vi "UI_1.vi"() -> (15 "Compressor  O/P":bool, 16 "Cond O/P":bool, 17 "Ev_Fan_1 O/P":bool, 18 "Ev_Fan_2 O/P":bool, 19 "Heater O/P":bool)   [LabVIEW 2017]
uses:
  Automatic_button.ctl
  Administration_button.ctl
  <vilib>/Utility/miscctls.llb/LVAnnotationListTypeDef.ctl
  admin_settings.vi
  <vilib>/Utility/file.llb/Write Delimited Spreadsheet (DBL).vi
  <vilib>/Utility/file.llb/Write Delimited Spreadsheet (string).vi
  <vilib>/Utility/NIReport.llb/NI_report.lvclass
  <resource>/objmgr/daqmx.rc
  <vilib>/Utility/NIReport.llb/Append Image to Report (path wrap).vi
  <vilib>/Utility/NIReport.llb/Append Text Table to Report (wrap).vi
panel:
  out "DevSerialNum 2":u32
  out "DevSerialNum":u32
  out "error out 6":errorcluster
  out "error out 11":errorcluster
  out "error out 10":errorcluster
  out "error out 9":errorcluster
  out "error out 8":errorcluster
  out "error out 7":errorcluster
  out "error out 4":errorcluster
  out "error out 3":errorcluster
  out "error out 5":errorcluster
  out "error out 2":errorcluster
  out "error out":errorcluster
  in  "Conrtols AUX 3":T1
  in  "Conrtols Valves 2":T2
  out "NI2":tag
  out "NI1":tag
  in  "Conrtols AUX 2":T1
  in  "Conrtols Valves":T2
  in  "Tab Control":enum32{"System", "Charts", "Faults"}(tab)
  out "Testing Mode":bool
  in  "Administration":T3
  in  "set point R":dbl
  in  "set point F":dbl
  in  "Auto":T4
  in  "Exit":bool
  out "T 9":dbl format="%#_3g"
  out "Segemnt_1.1 6":bool
  out "?":bool
  out "3.30":bool
  out "?":bool
  out "?":bool
  in  "Valve_8":bool
  in  "Valve_9":bool
  in  "Valve_10":bool
  out "T 4":dbl format="%#_3g"
  in  "Valve_2":bool
  out "P1":dbl format="%#_3g"
  out "T1":dbl format="%#_3g"
  out "S3.12":bool
  in  "Valve_11":bool
  out "T 10":dbl format="%#_3g"
  out "T 11":dbl format="%#_3g"
  out "P 3":dbl format="%#_3g"
  out "T 3":dbl format="%#_3g"
  out "S3.27":bool
  out "S3.23":bool
  out "S3.19":bool
  out "S3.28":bool
  out "S3.16":bool
  out "S3.18":bool
  out "?":bool
  out "OK Button 16":bool
  out "S3.15":bool
  out "?":bool
  out "?":bool
  out "?":bool
  out "Segment 1.4 5":bool
  out "?":bool
  out "?":bool
  in  "Ev_Fan_1":bool
  in  "Heater":bool
  in  "Valve_3":bool
  in  "Valve_4":bool
  in  "Valve_5":bool
  out "Segment_1":bool
  out "?":bool
  out "?":bool
  out "Segment_1 2":bool
  out "Segment 1.3":bool
  out "Segment 1.4":bool
  out "?":bool
  out "Segemnt_1.1 2":bool
  out "?":bool
  out "?":bool
  out "?":bool
  out "T 6":dbl format="%#_3g"
  out "?":bool
  out "OK Button":bool
  out "?":bool
  out "Segment 1.4 4":bool
  out "?":bool
  out "OK Button 3":bool
  out "Segemnt_1.1 3":bool
  out "?":bool
  out "OK Button 4":bool
  out "OK Button 5":bool
  out "OK Button 6":bool
  out "?":bool
  out "S3.37":bool
  out "S3.36":bool
  out "S3.35":bool
  out "Segment 1.4 7":bool
  out "?":bool
  out "?":bool
  in  "Ev_Fan_2":bool
  in  "Valve_6":bool
  in  "Valve_7":bool
  out "Segment_1 5":bool
  out "Segemnt_1.1 4":bool
  out "Segment_1 6":bool
  out "?":bool
  out "T 8":dbl format="%#_3g"
  out "?":bool
  out "Segemnt_1.1 5":bool
  out "?":bool
  out "?":bool
  out "?":bool
  out "T 7":dbl format="%#_3g"
  out "?":bool
  out "OK Button 11":bool
  out "?":bool
  out "Segment 1.4 8":bool
  out "?":bool
  out "OK Button 13":bool
  out "OK Button 15":bool
  out "?":bool
  out "P 4":dbl format="%#_3g"
  out "Segment_1 7":bool
  out "Segment_1 8":bool
  out "Segment_1 9":bool
  out "?":bool
  out "?":bool
  out "?":bool
  out "?":bool
  out "?":bool
  out "Segemnt_1.1 7":bool
  out "?":bool
  out "S3.1":bool
  out "S3.2":bool
  out "S3.3":bool
  out "S3.4":bool
  out "P5":dbl format="%#_3g"
  out "T5":dbl format="%#_3g"
  out "S3.6":bool
  out "S3.8":bool
  out "S3.11":bool
  out "S3.10":bool
  out "S3.9":bool
  out "S3.39":bool
  out "S3.38":bool
  out "?":bool
  out "3.34":bool
  out "3.33":bool
  out "3.32":bool
  out "?":bool
  out "3.31":bool
  out "?":bool
  out "S3.29":bool
  out "3.24":bool
  out "3.22":bool
  out "?":bool
  out "S3.25":bool
  out "3.21":bool
  out "3.20":bool
  out "Segment 1.4 2":bool
  out "Segment 1.4 3":bool
  in  "Cond":bool
  out "S3.14":bool
  out "S3.13":bool
  out "S3.17":bool
  in  "Valve_1":bool
  in  "Compressor":bool
  out "Segment 1.4 6":bool
  out "Segment 1.4 9":bool
  out "P 2":dbl format="%#_3g"
  out "T 2":dbl format="%#_3g"
  out "?":bool
  out "?":bool
  out "S3.25 2":bool
  out "?":bool
  out "S3.7":bool
  out "S3.5":bool
  in  "Save table":bool
  in  "Save image":bool
  in  "Tab Control 2":T5(tab)
  out "Cycle 1":string="6 ==> T11 , P11\n1 ==> T5 , P5\n2 ==> T1 , P1\n3 ==> T2 , P2\n4 ==> T9 , P2\n5 ==> T3 , P3"
  out "Cycle 2":string="6 ==> T11 , P11\n1 ==> T5 , P5\n2 ==> T1 , P1\n3 ==> T2 , P2\n4 ==> T9 , P2\n5 ==> T3 , P3"
  out "Cycle 3":string="6 ==> T11 , P11\n1 ==> T5 , P5\n2 ==> T1 , P1\n3 ==> T2 , P2\n4 ==> T9 , P2\n5 ==> T3 , P3"
  out "Cycle 4":string="9 ==> T10 , P10\n1 ==> T5 , P5\n2 ==> T1 , P1\n3 ==> T2 , P2\n7 ==> T8 , P2\n8 ==> T4 , P4"
  out "Cycle 5":string="9 ==> T10 , P10\n1 ==> T5 , P5\n2 ==> T1 , P1\n3 ==> T2 , P2\n7 ==> T8 , P2\n8 ==> T4 , P4"
  out "Cycle 6":string="9 ==> T10 , P10\n1 ==> T5 , P5\n2 ==> T1 , P1\n3 ==> T2 , P2\n7 ==> T8 , P2\n8 ==> T4 , P4"
  out "Cycle 7":string="1 ==> T5 , P5\n2 ==> T1 , P1\n3 ==> T2 , P2\n7 ==> T8 , P2\n8 ==> T4 , P4\n9 ==> T10 , P10\n\n4 ==> T9 , P2\n5 ==> T3 , P3\n6 ==> T11 , P11"
  out "Cycle 8":string="1 ==> T5 , P5\n2 ==> T1 , P1\n3 ==> T2 , P2\n7 ==> T8 , P2\n8 ==> T4 , P4\n9 ==> T10 , P10\n\n4 ==> T9 , P2\n5 ==> T3 , P3\n6 ==> T11 , P11"
  out "Cycle 9":string="1 ==> T5 , P5\n2 ==> T1 , P1\n3 ==> T2 , P2\n7 ==> T8 , P2\n8 ==> T4 , P4\n9 ==> T10 , P10\n\n4 ==> T9 , P2\n5 ==> T3 , P3\n6 ==> T11 , P11"
  out "Performance parameters":T6
  in  "Draw Points 2":bool
  out "Table":string[][](table)
  in  "Cycle":string(combo)="Cycle 1"
  in  "Draw Points":bool
  out "XY Graph":cluster{"all rows":dbl[], "all rows":dbl[]}[](graph)
  in  "m_dot_total":dbl=2.0 format="%#_13g"
  in  "m_dot_1":dbl=1.0 format="%#_13g"
  in  "m_dot_2":dbl=1.0 format="%#_13g"
  in  "h":dbl=372.0 format="%#_13g"
  in  "Valve 15 Fault":bool
  in  "Valve 13 Fault":bool
  in  "Valve 12 Fault":bool
  in  "Valve 11 Fault":bool
  # "TC"
  # "TC"
  # "Kg/s"
  # "KJ/Kg"
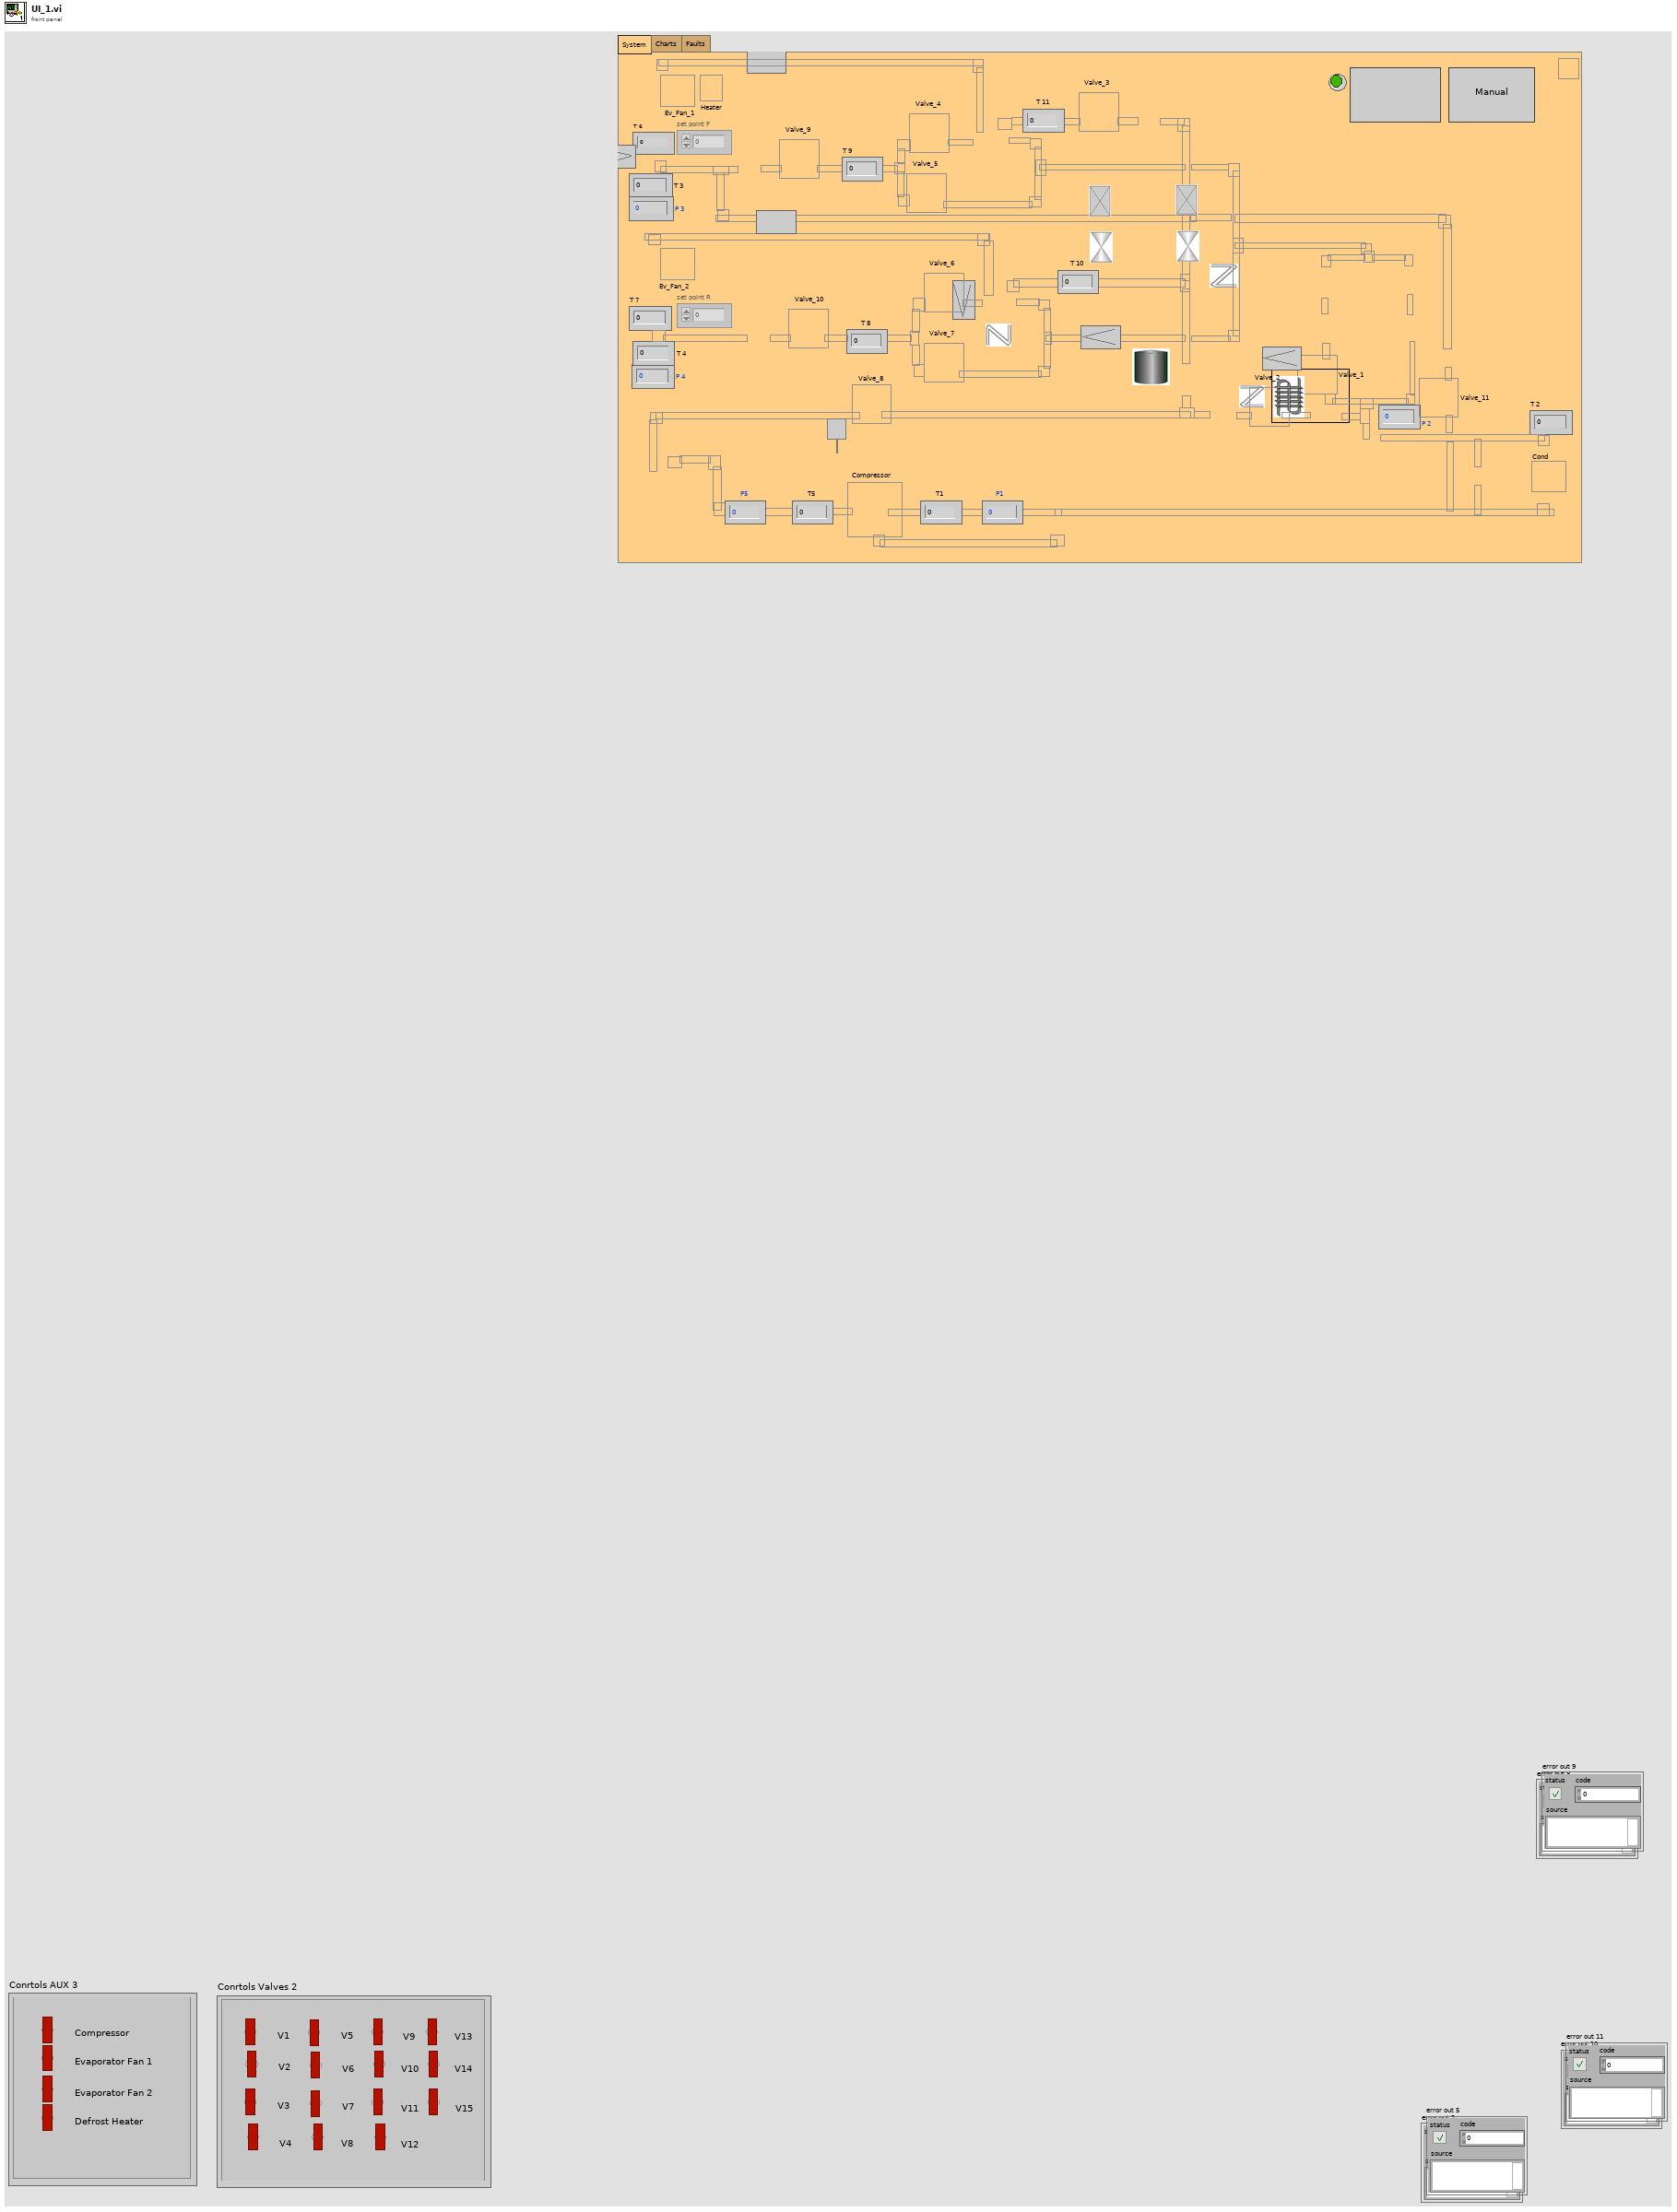
[diagram p1: front panel]
types:
  T1 = cluster{"Compressor":bool, "Evaporator Fan 1":bool, "Evaporator Fan 2":bool, "Defrost Heater":bool}
  T2 = cluster{"V1":bool, "V2":bool, "V3":bool, "V4":bool, "V5":bool, "V6":bool, "V7":bool, "V8":bool, "V9":bool, "V10":bool, "V11":bool, "V12":bool, "V13":bool, "V14":bool, "V15":bool}
  T3 = typedef "Administration_button.ctl" = bool
  T4 = typedef "Automatic_button.ctl" = bool
  T5 = enum32{"1", "2", "3", "4", "5", "6", "7", "8", "9"}
  T6 = cluster{"Condensation Capacity":dbl, "C.O.P  freez":dbl, "C.O.P  refrig":dbl}
  T7 = typedef "LVAnnotationListTypeDef.ctl" = cluster{"Name":string, "Color":u32, "Style":u8, "Point Style":u8, "Name Visible":bool, "Allow Drag":bool, "Annotation Mode":u32, "Plot":i32, "Index":i32, "Position":cluster{"X":dbl, "Y":dbl}, "X Scale":u32, "Y Scale":u32, "Show Arrow":bool, "Lock Name":bool, "Plot Area":i32, "Label Offset":cluster{"X":dbl, "Y":dbl}}[]
  T8 = enum16{"Standard Report", "HTML", "Word", "Excel"}
  T9 = enum8{"Enabled", "Disabled", "Disabled and Grayed Out"}
  T10 = cluster{"P1":dbl, "P2":dbl, "P3":dbl, "P4":dbl, "P5":dbl}
  T11 = cluster{"T1":dbl, "T2":dbl, "T3":dbl, "T4":dbl, "T5":dbl, "T6":dbl, "T7":dbl, "T8":dbl, "T9":dbl, "T10":dbl, "T11":dbl}
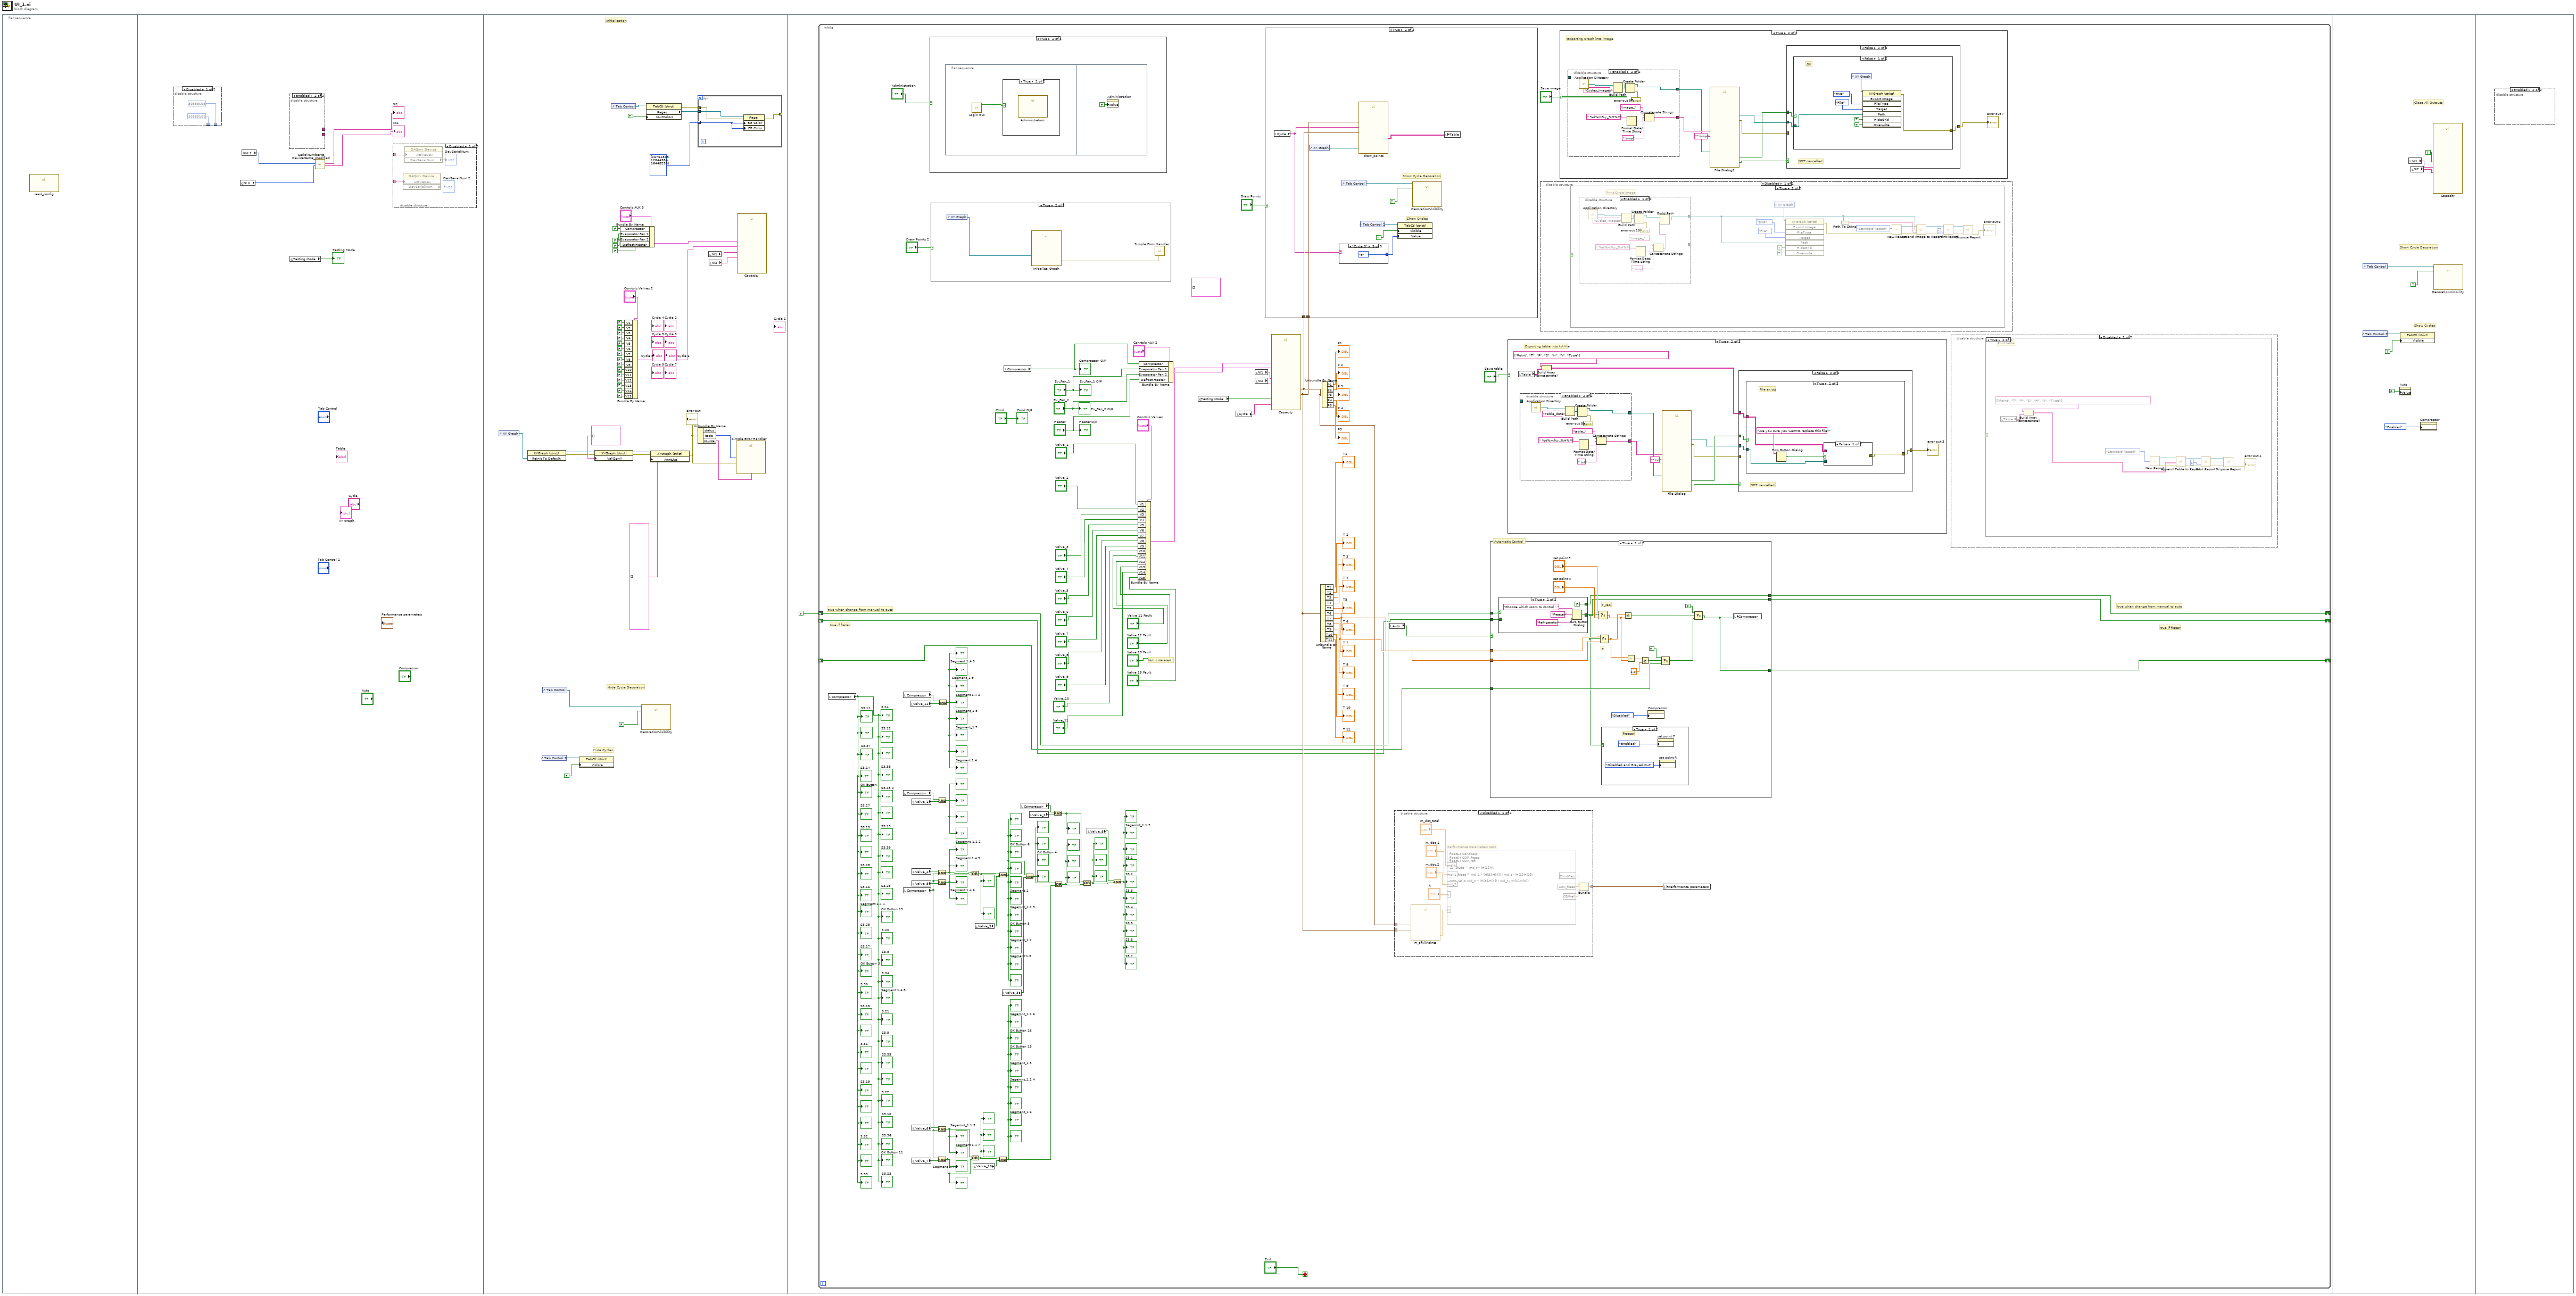
[diagram p0: block diagram]
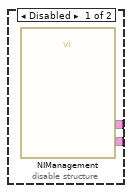
[diagram p4: hidden frame]
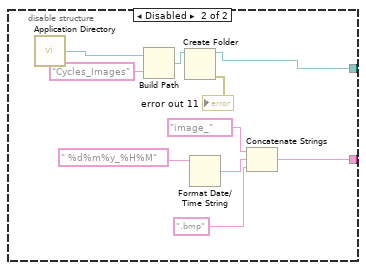
[diagram p8: hidden frame]
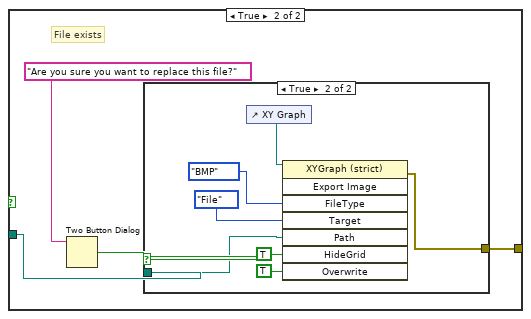
[diagram p14: hidden frame]
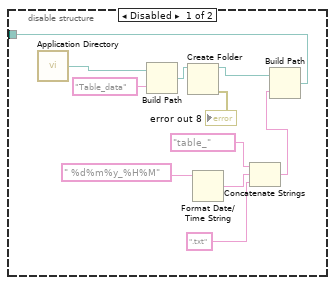
[diagram p16: hidden frame]
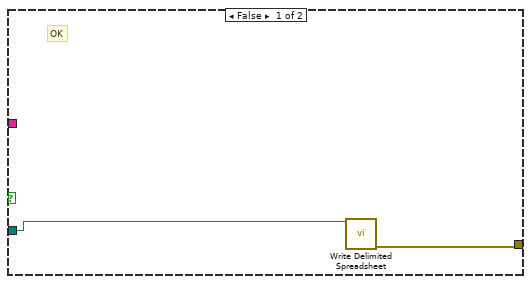
[diagram p19: hidden frame]
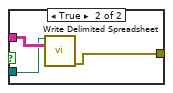
[diagram p20: hidden frame]
diagram:
  n1 = flat-sequence {
    frame #0 {
      n2 = call "read_config.vi"() -> ()  [unwired: 12 in]
    }
    frame #1 {
      n3 = disable-structure shown="Disabled" {
        disable-tunnel: [i64 30585608 ("NI1 Serial Number") _] -> _
        disable-tunnel: [i64 30585101 ("NI2 Serial Number") _] -> _
        frame Disabled {
        }
        frame Enabled {
        }
      }
      n4 = global read "admin_settings.vi" "NI 2"() -> (w3:i64)
      n5 = global read "admin_settings.vi" "NI 1"() -> (w4:i64)
      n6 = disable-structure shown="Enabled" {
        disable-tunnel: [w13 _] -> _
        disable-tunnel: [w12 _] -> _
        frame Disabled {
          n7 = call "NIManagement.vi"() -> ("NI2"=w12:tag, "NI1"=w13:tag)  [unwired: 8 in, 2 out]
        }
        frame Enabled {
        }
      }
      n8 = global read "admin_settings.vi" "Testing Mode"() -> (→"Testing Mode":bool)
      n9 = call "SerialNumber to DeviceName_modified.vi"("NI2 Serial Number"=w3, "NI1 Serial Number"=w4) -> ("NI2 Device Name"=→"NI2":tag, "NI1 Device Name"=→"NI1":tag)  [unwired: 7 in, 1 out]
      n10 = disable-structure shown="Disabled" {
        disable-tunnel: _ -> [w7 _]
        disable-tunnel: _ -> [w6 _]
        frame Disabled {
          n11 = property class="DAQmx Device"("ActiveDev"=w6) -> ("DevSerialNum"=→"DevSerialNum 2":u32)  [unwired: 2 in, 2 out]
          n12 = property class="DAQmx Device"("ActiveDev"=w7) -> ("DevSerialNum"=→"DevSerialNum":u32)  [unwired: 2 in, 2 out]
        }
        frame Enabled {
        }
      }
    }
    frame #2 {
      # "Hide Cycles"
      # "Hide Cycle Decoration"
      # "Initialization"
      n13 = control-ref of="XY Graph"() -> (w20:refnum<vi>)
      n14 = invoke class="XYGraph (strict)" method="Reinit To Default"(reference=w20) -> (reference out=w26:refnum<vi>, error out=w17:errorcluster)  [unwired: 2 in, 1 out]
      n15 = control-ref of="Tab Control 2"() -> (w15:refnum<vi>)
      n16 = control-ref of="Tab Control"() -> (w19:refnum<vi>)
      n17 = property class="TabCtl (strict)"(reference=w15, "Visible"=FALSE) -> ()  [unwired: 1 in, 2 out]
      n18 = property class="XYGraph (strict)"(reference=w26, error in=w17, "Val(Sgnl)"=cluster{"all rows":dbl[], "all rows":dbl[]}[] [] ("Value (Signaling)")) -> (reference out=w25:refnum<vi>, error out=w23:errorcluster)
      n19 = control-ref of="Tab Control"() -> (w28:refnum<vi>)
      n20 = Bundle By Name(cluster="Conrtols AUX 3", "Compressor"=FALSE, "Evaporator Fan 1"=FALSE, "Evaporator Fan 2"=FALSE, "Defrost Heater"=FALSE) -> (w36:T1)
      n21 = Bundle By Name(cluster="Conrtols Valves 2", "V1"=FALSE, "V2"=FALSE, "V3"=FALSE, "V4"=FALSE, "V5"=FALSE, "V6"=FALSE, "V7"=FALSE, "V8"=FALSE, "V9"=FALSE, "V10"=FALSE, "V11"=FALSE, "V12"=FALSE, "V13"=FALSE, "V14"=FALSE, "V15"=FALSE) -> (w35:T2)
      n22 = call "DecorationVisibility.vi"("Visible"=FALSE, "TabControl in"=w19) -> ()  [unwired: 9 in, 1 out]
      n23 = property class="TabCtl (strict)"(reference=w28, "MultColors"=TRUE ("Mehrere Farben zulassen")) -> (error out=w30:errorcluster, "Pages"=w32:refnum<vi>[])  [unwired: 1 in, 1 out]
      n24 = property on="Property Node" class="XYGraph (strict)"(reference=w25, error in=w23, "AnntList"=T7 [] ("Annotation List")) -> (error out=w18:errorcluster)  [unwired: 1 out]
      "error out" <- w18
      n25 = for {
        tunnel: w32 -> [w61] mode=indexing
        tunnel: u32[] [16764808, 12844984, 16448250] -> [w60] mode=indexing
        tunnel: w30 -> [w59]
        tunnel: [w58] -> _ mode=indexing
        n26 = property class="Page"(reference=w61, error in=w59, "BG Color"=w60, "FG Color"=w60) -> (error out=w58:errorcluster)  [unwired: 1 out]
      }
      n27 = Unbundle By Name(w18) -> ("code"=w21:i32, "source"=w22:string)  [unwired: 1 out]
      n28 = local read "NI1"() -> (w34:tag)
      n29 = local read "NI2"() -> (w33:tag)
      n30 = call <vilib>:"Simple Error Handler.vi"("error code (no error:0)"=w21, "error source (\" \")"=w22, "error in (no error)"=w18) -> ()  [unwired: 2 in, 5 out]
      n31 = call "Capacity.vi"("Conrtols Valves"=w35, "Conrtols AUX"=w36, "NI1"=w34, "NI2"=w33) -> ()  [unwired: 10 in, 2 out]
    }
    frame #3 {
      n32 = while {
        shift-right: [w74] -> _
        shift-left: _ -> [w73]
        shift-right: [w70] -> _
        shift-left: TRUE -> [w71]
        shift-right: [w69] -> _
        shift-left: _ -> [w68]
        stop <- "Exit" stop-if-true
        (unwired) cluster{"all rows":dbl[], "all rows":dbl[]}[] [] ("Output Graphs")
        # "Automatic Control"
        # "true when change from manual to auto"
        # "true if frezer"
        # "true when change from manual to auto"
        # "true if frezer"
        # "Not is deleted !"
        n33 = local read "Compressor"() -> (→"S3.8" →"S3.9" →"S3.10" →"S3.11" →"S3.15" →"S3.19" →"S3.14" →"S3.16" →"S3.17" →"S3.18" →"S3.13" →"S3.12" →"3.22" →"S3.25 2" →"S3.23" →"3.21" →"3.20" →"S3.25" →"S3.29" →"3.33" →"3.30" →"S3.27" →"S3.28" →"3.34" →"?" →"S3.35" →"S3.39" →"S3.38" →"S3.37" →"3.32" →"S3.36" →"3.24" →"3.31" →"?" →"?" →"?" →"OK Button" →"?" →"Segment 1.4 4" →"?" →"OK Button 3" →"?" →"?" →"?" →"?" →"OK Button 13" →"Segment 1.4 8" →"OK Button 11" →"?":bool)
        n34 = local read "Compressor"() -> (w150:bool)
        n35 = local read "Compressor"() -> (w151:bool)
        n36 = local read "Compressor"() -> (w137:bool)
        n37 = local read "Valve_11"() -> (w149:bool)
        n38 = local read "Valve_1"() -> (w152:bool)
        n39 = local read "Valve_4"() -> (w145:bool)
        n40 = local read "Valve_5"() -> (w144:bool)
        n41 = local read "Valve_6"() -> (w139:bool)
        n42 = local read "Valve_7"() -> (w138:bool)
        n43 = case shown="True" "Administration" {
          frame False {
          }
          frame True {
            n44 = flat-sequence {
              frame #0 {
                n45 = call "Login GUI.vi"() -> ("true"=w154:bool)  [unwired: 11 in]
                n46 = case shown="True" w154 {
                  frame False {
                  }
                  frame True {
                    n47 = call "Administration.vi"() -> ()  [unwired: 12 in]
                  }
                }
              }
              frame #1 {
                n48 = property on="Administration" class="Bool (strict)"("Value"=T3 FALSE ("Administration")) -> ()  [unwired: 2 in, 2 out]
              }
            }
          }
        }
        n49 = case shown="True" "Draw Points 2" {
          frame False {
          }
          frame True {
            n50 = control-ref of="XY Graph"() -> (w354:refnum<vi>)
            n51 = call "Initialize_Graph.vi"("XYGraph in"=w354) -> ("error out"=w353:errorcluster)  [unwired: 10 in]
            n52 = call <vilib>:"Simple Error Handler.vi"("error in (no error)"=w353) -> ()  [unwired: 4 in, 5 out]
          }
        }
        n53 = And(x=w145, y=w137) -> (x .and. y?=w147:bool)
        "Segemnt_1.1 2" <- w147
        "Segment 1.4 5" <- w147
        n54 = And(x=w137, y=w144) -> (x .and. y?=w146:bool)
        "?" <- w146
        "Segment 1.4 6" <- w146
        n55 = And(x=w139, y=w137) -> (x .and. y?=w136:bool)
        "Segemnt_1.1 5" <- w136
        "Segment 1.4 7" <- w136
        n56 = And(x=w137, y=w138) -> (x .and. y?=w135:bool)
        "?" <- w135
        "Segment 1.4 9" <- w135
        n57 = And(x=w151, y=w152) -> (x .and. y?=→"?" →"?" →"?" →"?":bool)
        n58 = And(x=w150, y=w149) -> (x .and. y?=→"Segment 1.4" →"?" →"Segment_1 7" →"Segment_1 8" →"Segment_1 9" →"?" →"Segment 1.4 2" →"Segment 1.4 3":bool)
        n59 = Or(x=w147, y=w146) -> (x .or. y?=w142:bool)
        "?" <- w142
        "?" <- w142
        n60 = Or(x=w136, y=w135) -> (x .or. y?=w133:bool)
        "?" <- w133
        "?" <- w133
        "?" <- w133
        n61 = local read "Valve_10"() -> (w134:bool)
        n62 = local read "Valve_9"() -> (w143:bool)
        n63 = And(x=w142, y=w143) -> (x .and. y?=w141:bool)
        "?" <- w141
        "Segment_1" <- w141
        "?" <- w141
        "?" <- w141
        "Segment_1 2" <- w141
        "Segment 1.3" <- w141
        "Segemnt_1.1 3" <- w141
        "?" <- w141
        "?" <- w141
        "OK Button 5" <- w141
        "OK Button 6" <- w141
        n64 = And(x=w133, y=w134) -> (x .and. y?=w126:bool)
        "?" <- w126
        "?" <- w126
        "Segment_1 5" <- w126
        "Segemnt_1.1 4" <- w126
        "?" <- w126
        "Segment_1 6" <- w126
        "Segemnt_1.1 6" <- w126
        "OK Button 15" <- w126
        "OK Button 16" <- w126
        n65 = local read "Valve_3"() -> (w140:bool)
        n66 = local read "Compressor"() -> (w72:bool)
        "Compressor  O/P" <- w72
        n67 = local read "Compressor"() -> (w129:bool)
        n68 = And(x=w141, y=w140) -> (x .and. y?=w132:bool)
        "?" <- w132
        "?" <- w132
        "OK Button 4" <- w132
        "?" <- w132
        n69 = local read "Valve_2"() -> (w128:bool)
        n70 = And(x=w129, y=w128) -> (x .and. y?=w125:bool)
        "?" <- w125
        n71 = Or(x=w132, y=w126) -> (x .or. y?=w130:bool)
        "?" <- w130
        "?" <- w130
        "?" <- w130
        n72 = Or(x=w125, y=w130) -> (x .or. y?=w124:bool)
        "?" <- w124
        "?" <- w124
        "?" <- w124
        n73 = local read "Valve_8"() -> (w127:bool)
        n74 = And(x=w127, y=w124) -> (x .and. y?=→"S3.1" →"S3.2" →"S3.3" →"S3.4" →"S3.6" →"S3.5" →"S3.7" →"?" →"Segemnt_1.1 7" →"?":bool)
        n75 = Bundle By Name(cluster="Conrtols Valves", "V1"="Valve_1", "V2"="Valve_2", "V3"="Valve_3", "V4"="Valve_4", "V5"="Valve_5", "V6"="Valve_6", "V7"="Valve_7", "V8"="Valve_8", "V9"="Valve_9", "V10"="Valve_10", "V11"="Valve 11 Fault", "V12"="Valve 12 Fault", "V13"="Valve 13 Fault", "V14"="Valve_11", "V15"="Valve 15 Fault") -> (w85:T2)
        n76 = Bundle By Name(cluster="Conrtols AUX 2", "Compressor"=w72, "Evaporator Fan 1"="Ev_Fan_1", "Evaporator Fan 2"="Ev_Fan_2", "Defrost Heater"="Heater") -> (w86:T1)
        n77 = global read "admin_settings.vi" "Testing Mode"() -> (w64:bool)
        n78 = local read "Cycle"() -> (w67:string)
        n79 = local read "NI1"() -> (w84:tag)
        n80 = local read "NI2"() -> (w83:tag)
        n81 = call "Capacity.vi"("Conrtols Valves"=w85, "Testing"=w64, "Cycle"=w67, "Conrtols AUX"=w86, "NI1"=w84, "NI2"=w83) -> ("Pressure Sensors 2"=w81:T10, "Temperature Sensors"=w80:T11)  [unwired: 8 in]
        n82 = case shown="True" "Draw Points" {
          tunnel: w81 -> [_ w364]
          tunnel: w80 -> [_ w363]
          frame False {
          }
          frame True {
            # "Show Cycles"
            # "Show Cycle Decoration"
            n83 = local read "Cycle"() -> (w357:string)
            n84 = control-ref of="XY Graph"() -> (w356:refnum<vi>)
            n85 = case shown="\"Cycle 9\"" w357 {
              tunnel: [T5."1" ("Value") T5."2" ("Value") T5."3" ("Value") T5."4" ("Value") T5."5" ("Value") T5."6" ("Value") T5."7" ("Value") T5."8" ("Value") T5."9" ("Value")] -> w358
              frame "Cycle 1", Default {
              }
              frame "Cycle 2" {
              }
              frame "Cycle 3" {
              }
              frame "Cycle 4" {
              }
              frame "Cycle 5" {
              }
              frame "Cycle 6" {
              }
              frame "Cycle 7" {
              }
              frame "Cycle 8" {
              }
              frame "Cycle 9" {
              }
            }
            n86 = control-ref of="Tab Control"() -> (w361:refnum<vi>)
            n87 = call "draw_points.vi"("XY Graph Ref In"=w356, "Cycle"=w357, "T cluster"=w363, "P cluster"=w364) -> ("Table"=w355:string[][])  [unwired: 6 in, 1 out]
            n88 = control-ref of="Tab Control 2"() -> (w362:refnum<vi>)
            n89 = property class="TabCtl (strict)"(reference=w362, "Visible"=TRUE, "Value"=w358) -> ()  [unwired: 1 in, 2 out]
            n90 = call "DecorationVisibility.vi"("Visible"=TRUE, "TabControl in"=w361) -> ()  [unwired: 9 in, 1 out]
            n91 = local write "Table"(w355) -> ()
          }
        }
        n92 = Unbundle By Name(w80) -> ("T1"=→"T1":dbl, "T2"=→"T 2":dbl, "T3"=→"T 3":dbl, "T4"=→"T 4":dbl, "T5"=→"T5":dbl, "T6"=w76:dbl, "T7"=w75:dbl, "T8"=→"T 8":dbl, "T9"=→"T 9":dbl, "T10"=→"T 10":dbl, "T11"=→"T 11":dbl)
        "T 6" <- w76
        "T 7" <- w75
        n93 = Unbundle By Name(w81) -> ("P1"=→"P1":dbl, "P2"=→"P 2":dbl, "P3"=→"P 3":dbl, "P4"=→"P 4":dbl, "P5"=→"P5":dbl)
        n94 = local read "Auto"() -> (w77:T4)
        n95 = disable-structure shown="Disabled" {
          disable-tunnel: w81 -> [w316 _]
          disable-tunnel: w80 -> [w315 _]
          disable-tunnel: [w306 _] -> w79
          frame Disabled {
            # "Performance Parameters Calc."
            n96 = call "H_ofAllPoints.vi"("Temperature Sensors"=w315, "Pressure Sensors in"=w316) -> ("H's"=w310:dbl[])  [unwired: 9 in]
            n97 = formula code="float64 CondCap;\nfloat64 COP_freez;\nfloat64 COP_ref;\n\nCondCap = md_t * (H[1]-h);\n\nCOP_freez = md_1 * (H[5]-H[4]) / md_t / (H[1]-H[0]);\n\nCOP_ref = md_2 * (H[8]-H[7]) / md_t / (H[1]-H[0]);"("md_t"="m_dot_total", "md_1"="m_dot_1", "md_2"="m_dot_2", "h"="h", "H"=w310) -> ("CondCap"=w309:dbl, "COP_freez"=w308:dbl, "COPref"=w307:dbl)
            n98 = Bundle(w309, w308, "COPref"=w307) -> (w306:cluster{dbl, dbl, "COPref":dbl})  [unwired: 1 in]
          }
          frame Enabled {
          }
        }
        n99 = case shown="True" w77 {
          tunnel: w76 -> [_ w339]
          tunnel: w75 -> [_ w338]
          tunnel: [w321 w327] -> w74
          tunnel: w73 -> [_ w333]
          tunnel: w71 -> [_ w325]
          tunnel: [w320 w324] -> w70
          tunnel: [w320 w322] -> w69
          tunnel: w68 -> [_ w323]
          frame False {
            w320 = TRUE
            n100 = property on="Compressor" class="Bool (strict)"("DisabledEnum"=T9."Enabled" ("Disabled")) -> ()  [unwired: 2 in, 2 out]
            n101 = property on="set point F" class="DigNum (strict)"("DisabledEnum"=T9."Disabled and Grayed Out" ("Disabled")) -> ()  [unwired: 2 in, 2 out]
            n102 = property on="set point R" class="DigNum (strict)"("DisabledEnum"=T9."Disabled and Grayed Out" ("Disabled")) -> ()  [unwired: 2 in, 2 out]
            n103 = local read "Compressor"() -> (w321:bool)
          }
          frame True {
            # "T_req"
            # "T"
            n104 = case shown="True" w325 {
              tunnel: [w346 w349] -> w322
              tunnel: [FALSE FALSE] -> w324
              tunnel: w323 -> [w346 _]
              frame False {
              }
              frame True {
                n105 = Two Button Dialog(message="Choose which room to control : ", 1:"Refrigerator" ("F button name (\"Cancel\")"), 2:"Freezer" ("T button name (\"OK\")")) -> (T button?=w349:bool)
              }
            }
            n106 = Select(t="set point F", s=w322, f="set point R") -> (s? t:f=w329:dbl)
            n107 = Select(t=w339, s=w322, f=w338) -> (s? t:f=w330:dbl)
            n108 = case shown="True" w322 {
              frame True {
                # "freezer"
                n109 = property on="set point F" class="DigNum (strict)"("DisabledEnum"=T9."Enabled" ("Disabled")) -> ()  [unwired: 2 in, 2 out]
                n110 = property on="set point R" class="DigNum (strict)"("DisabledEnum"=T9."Disabled and Grayed Out" ("Disabled")) -> ()  [unwired: 2 in, 2 out]
              }
              frame False {
                # "Refrig."
                n111 = property on="set point R" class="DigNum (strict)"("DisabledEnum"=T9."Enabled" ("Disabled")) -> ()  [unwired: 2 in, 2 out]
                n112 = property on="set point F" class="DigNum (strict)"("DisabledEnum"=T9."Disabled and Grayed Out" ("Disabled")) -> ()  [unwired: 2 in, 2 out]
              }
            }
            n113 = Less Or Equal?(x=w330, y=w329) -> (x <= y?=w332:bool)
            n114 = Subtract(x=w330, y=w329) -> (x-y=w337:dbl)
            n115 = Greater Or Equal?(x=w337, y=1.0) -> (x >= y?=w335:bool)
            n116 = property on="Compressor" class="Bool (strict)"("DisabledEnum"=T9."Disabled" ("Disabled")) -> ()  [unwired: 2 in, 2 out]
            n117 = Select(t=TRUE, s=w335, f=w333) -> (s? t:f=w328:bool)
            n118 = Select(t=FALSE, s=w332, f=w328) -> (s? t:f=w327:bool)
            n119 = local write "Compressor"(w327) -> ()
          }
        }
        n120 = case shown="True" "Save table" {
          frame False {
          }
          frame True {
            # "Exporting table into txt file"
            n121 = local read "Table"() -> (w269:string[][])
            n122 = disable-structure shown="Enabled" {
              disable-tunnel: [w286 _] -> _
              disable-tunnel: [_ w297] -> w267
              disable-tunnel: [_ w296] -> w266
              frame Disabled {
                n123 = call <vilib>:"Application Directory.vi"() -> ("Application Directory"=w291:path)
                n124 = Build Path(base path=w291, name or relative path="Table_data") -> (appended path=w289:path)
                n125 = Create Folder(path (use dialog)=w289) -> (created path=w288:path, error out=→"error out 2":errorcluster)  [unwired: 2 in, 1 out]
                n126 = Format Date/Time String(time format string (%c)=" %d%m%y_%H%M") -> (date/time string=w292:string)  [unwired: 2 in]
                n127 = Concatenate Strings("table_" ("name or relative path"), w292, ".txt" ("string")) -> (w294:string)
                n128 = Build Path(base path=w288, name or relative path=w294) -> (appended path=w286:path)
              }
              frame Enabled {
                n129 = call <vilib>:"Application Directory.vi"() -> ("Application Directory"=w302:path)
                n130 = Build Path(base path=w302, name or relative path="Table_data") -> (appended path=w300:path)
                n131 = Create Folder(path (use dialog)=w300) -> (created path=w297:path, error out=→"error out 5":errorcluster)  [unwired: 2 in, 1 out]
                n132 = Format Date/Time String(time format string (%c)=" %d%m%y_%H%M") -> (date/time string=w303:string)  [unwired: 2 in]
                n133 = Concatenate Strings("table_" ("name or relative path"), w303, ".txt" ("string")) -> (w296:string)
              }
            }
            n134 = Build Array (concatenate)(string[] ["Point", "T", "P", "S", "H", "V", "Type"], w269) -> (w262:string[][])
            n135 = call "File Dialog"("start path"=w267, "default name"=w266, "pattern (all files)"="*.txt") -> ("selected path"=w263:path, "exists"=w264:bool, "cancelled"=w260:bool, "error out"=w259:errorcluster)  [unwired: 9 in]
            n136 = case shown="False" w260 {
              tunnel: w264 -> [_ w274]
              tunnel: w263 -> [_ w273]
              tunnel: w262 -> [_ w272]
              tunnel: [w270 w271] -> w261
              tunnel: w259 -> [w270 _]
              frame True {
                # "Cancelled"
              }
              frame False {
                # "NOT cancelled"
                n137 = case shown="True" w274 {
                  tunnel: w273 -> [w276 w278]
                  tunnel: w272 -> [_ w279]
                  tunnel: [w275 w277] -> w271
                  frame False {
                    # "OK"
                    n138 = call-poly <vilib>:"Write Delimited Spreadsheet.vi"("file path (dialog if empty)"=w276) -> ("error out"=w275:errorcluster)  [unwired: 13 in, 1 out]
                  }
                  frame True {
                    # "File exists"
                    n139 = Two Button Dialog(message="Are you sure you want to replace this file?") -> (T button?=w280:bool)  [unwired: 2 in]
                    n140 = case shown="False" w280 {
                      tunnel: w279 -> [_ w284]
                      tunnel: w278 -> [_ w283]
                      tunnel: [_ w282] -> w277
                      frame False {
                      }
                      frame True {
                        n141 = call-poly <vilib>:"Write Delimited Spreadsheet.vi"("file path (dialog if empty)"=w283, "2D data"=w284) -> ("error out"=w282:errorcluster)  [unwired: 12 in, 1 out]
                      }
                    }
                  }
                }
              }
            }
            "error out 3" <- w261
          }
        }
        n142 = disable-structure shown="Disabled" {
          frame Disabled {
            n143 = case shown="True" w156 {
              frame False {
              }
              frame True {
                # "Print Cycle image"
                n144 = disable-structure shown="Enabled" {
                  disable-tunnel: [w174 w186] -> w158
                  disable-tunnel: [_ w185] -> _
                  frame Enabled {
                    n145 = call <vilib>:"Application Directory.vi"() -> ("Application Directory"=w180:path)
                    n146 = Build Path(base path=w180, name or relative path="Cycles_Images") -> (appended path=w178:path)
                    n147 = Create Folder(path (use dialog)=w178) -> (created path=w177:path, error out=→"error out 10":errorcluster)  [unwired: 2 in, 1 out]
                    n148 = Format Date/Time String(time format string (%c)=" %d%m%y_%H%M") -> (date/time string=w181:string)  [unwired: 2 in]
                    n149 = Concatenate Strings("image_" ("name or relative path"), w181, ".bmp" ("string")) -> (w183:string)
                    n150 = Build Path(base path=w177, name or relative path=w183) -> (appended path=w174:path)
                  }
                  frame Disabled {
                    n151 = call <vilib>:"Application Directory.vi"() -> ("Application Directory"=w191:path)
                    n152 = Build Path(base path=w191, name or relative path="Cycles_Images") -> (appended path=w189:path)
                    n153 = Create Folder(path (use dialog)=w189) -> (created path=w186:path, error out=→"error out 11":errorcluster)  [unwired: 2 in, 1 out]
                    n154 = Format Date/Time String(time format string (%c)=" %d%m%y_%H%M") -> (date/time string=w192:string)  [unwired: 2 in]
                    n155 = Concatenate Strings("image_" ("name or relative path"), w192, ".bmp" ("string")) -> (w185:string)
                  }
                }
                n156 = control-ref of="XY Graph"() -> (w160:refnum<vi>)
                n157 = invoke class="XYGraph (strict)" method="Export Image"(reference=w160, "FileType"=enum32{"BMP", "EPS", "EMF", "PICT"}."BMP" ("File Type"), "Target"=enum32{"File", "Clipboard"}."File", "Path"=w158, "HideGrid"=TRUE ("Hide Grid"), "Overwrite"=TRUE ("Always Overwrite")) -> (error out=w159:errorcluster)  [unwired: 2 in, 7 out]
                n158 = Path To String(path=w158) -> (string=w168:string)
                n159 = call <vilib>:"New Report.vi"("report type"=enum16{"Standard Report", "HTML"}."Standard Report", "error in (no error)"=w159) -> ("report out"=w166:refnum<class "NI_report.lvclass">, "error out"=w167:errorcluster)  [unwired: 12 in]
                n160 = call-poly <vilib>:"Append Image to Report.vi"("report in"=w166, "path or URL of image"=w158, "caption or alternative string"=w168, "error in (no error)"=w167) -> ("report out"=w169:refnum<class "NI_report.lvclass">, "error out"=w171:errorcluster)  [unwired: 8 in, 2 out]
                n161 = call-dynamic "Print Report.vi"("report in"=w169, "number of copies (1)"=1, "error in (no error)"=w171) -> ("report out"=w172:refnum<class "NI_report.lvclass">, "error out"=w173:errorcluster)  [unwired: 11 in]
                n162 = call-dynamic "Dispose Report.vi"("report in"=w172, "error in (no error)"=w173) -> ("error out"=→"error out 6":errorcluster)  [unwired: 13 in]
              }
            }
          }
          frame Enabled {
          }
        }
        n163 = case shown="True" "Save image" {
          frame False {
          }
          frame True {
            # "Exporting Graph into image"
            n164 = disable-structure shown="Enabled" {
              disable-tunnel: [w239 _] -> _
              disable-tunnel: [_ w250] -> w209
              disable-tunnel: [_ w249] -> w210
              frame Disabled {
                n165 = call <vilib>:"Application Directory.vi"() -> ("Application Directory"=w244:path)
                n166 = Build Path(base path=w244, name or relative path="Table_data") -> (appended path=w242:path)
                n167 = Create Folder(path (use dialog)=w242) -> (created path=w241:path, error out=→"error out 8":errorcluster)  [unwired: 2 in, 1 out]
                n168 = Format Date/Time String(time format string (%c)=" %d%m%y_%H%M") -> (date/time string=w245:string)  [unwired: 2 in]
                n169 = Concatenate Strings("table_" ("name or relative path"), w245, ".txt" ("string")) -> (w247:string)
                n170 = Build Path(base path=w241, name or relative path=w247) -> (appended path=w239:path)
              }
              frame Enabled {
                n171 = call <vilib>:"Application Directory.vi"() -> ("Application Directory"=w255:path)
                n172 = Build Path(base path=w255, name or relative path="Cycles_Images") -> (appended path=w253:path)
                n173 = Create Folder(path (use dialog)=w253) -> (created path=w250:path, error out=→"error out 9":errorcluster)  [unwired: 2 in, 1 out]
                n174 = Format Date/Time String(time format string (%c)=" %d%m%y_%H%M") -> (date/time string=w256:string)  [unwired: 2 in]
                n175 = Concatenate Strings("image_" ("name or relative path"), w256, ".bmp" ("string")) -> (w249:string)
              }
            }
            n176 = call "File Dialog2"("start path"=w209, "default name"=w210, "pattern (all files)"="*.bmp") -> ("selected path"=w213:path, "exists"=w212:bool, "cancelled"=w214:bool, "error out"=w215:errorcluster)  [unwired: 9 in]
            n177 = case shown="False" w214 {
              tunnel: w212 -> [_ w219]
              tunnel: w213 -> [_ w218]
              tunnel: [w216 w217] -> w208
              tunnel: w215 -> [w216 _]
              frame True {
                # "Cancelled"
              }
              frame False {
                # "NOT cancelled"
                n178 = case shown="False" w219 {
                  tunnel: w218 -> [w221 w228]
                  tunnel: [w220 w227] -> w217
                  frame False {
                    # "OK"
                    n179 = control-ref of="XY Graph"() -> (w226:refnum<vi>)
                    n180 = invoke class="XYGraph (strict)" method="Export Image"(reference=w226, "FileType"=enum32{"BMP", "EPS", "EMF", "PICT"}."BMP" ("File Type"), "Target"=enum32{"File", "Clipboard"}."File", "Path"=w221, "HideGrid"=TRUE ("Hide Grid"), "Overwrite"=TRUE ("Always Overwrite")) -> (error out=w220:errorcluster)  [unwired: 2 in, 7 out]
                  }
                  frame True {
                    # "File exists"
                    n181 = Two Button Dialog(message="Are you sure you want to replace this file?") -> (T button?=w229:bool)  [unwired: 2 in]
                    n182 = case shown="True" w229 {
                      tunnel: w228 -> [_ w232]
                      tunnel: [_ w231] -> w227
                      frame False {
                      }
                      frame True {
                        n183 = control-ref of="XY Graph"() -> (w237:refnum<vi>)
                        n184 = invoke class="XYGraph (strict)" method="Export Image"(reference=w237, "FileType"=enum32{"BMP", "EPS", "EMF", "PICT"}."BMP" ("File Type"), "Target"=enum32{"File", "Clipboard"}."File", "Path"=w232, "HideGrid"=TRUE ("Hide Grid"), "Overwrite"=TRUE ("Always Overwrite")) -> (error out=w231:errorcluster)  [unwired: 2 in, 7 out]
                      }
                    }
                  }
                }
              }
            }
            "error out 7" <- w208
          }
        }
        n185 = local write "Performance parameters"(w79) -> ()
        n186 = disable-structure shown="Disabled" {
          frame Disabled {
            n187 = case shown="True" w195 {
              frame False {
              }
              frame True {
                # "Print table"
                n188 = local read "Table"() -> (w197:string[][])
                n189 = Build Array (concatenate)(string[] ["Point", "T", "P", "S", "H", "V", "Type"], w197) -> (w196:string[][])
                n190 = call <vilib>:"New Report.vi"("report type"=T8."Standard Report") -> ("report out"=w201:refnum<class "NI_report.lvclass">, "error out"=w199:errorcluster)  [unwired: 13 in]
                n191 = call-poly <vilib>:"Append Table to Report.vi"("report in"=w201, "text data"=w196, "error in (no error)"=w199) -> ("report out"=w207:refnum<class "NI_report.lvclass">, "error out"=w206:errorcluster)  [unwired: 9 in, 2 out]
                n192 = call-dynamic "Print Report.vi"("report in"=w207, "number of copies (1)"=1, "error in (no error)"=w206) -> ("report out"=w204:refnum<class "NI_report.lvclass">, "error out"=w203:errorcluster)  [unwired: 11 in]
                n193 = call-dynamic "Dispose Report.vi"("report in"=w204, "error in (no error)"=w203) -> ("error out"=→"error out 4":errorcluster)  [unwired: 13 in]
              }
            }
          }
          frame Enabled {
          }
        }
        "Heater O/P" <- "Heater"
        "Ev_Fan_1 O/P" <- "Ev_Fan_1"
        "Ev_Fan_2 O/P" <- "Ev_Fan_2"
        "Cond O/P" <- "Cond"
      }
    }
    frame #4 {
      # "Show Cycles"
      # "Show Cycle Decoration"
      # "Close All Outputs"
      n194 = control-ref of="Tab Control"() -> (w377:refnum<vi>)
      n195 = control-ref of="Tab Control 2"() -> (w379:refnum<vi>)
      n196 = property on="Auto" class="Bool (strict)"("Value"=FALSE) -> ()  [unwired: 2 in, 2 out]
      n197 = property class="TabCtl (strict)"(reference=w379, "Visible"=TRUE) -> ()  [unwired: 1 in, 2 out]
      n198 = local read "NI1"() -> (w382:tag)
      n199 = local read "NI2"() -> (w381:tag)
      n200 = property on="Compressor" class="Bool (strict)"("DisabledEnum"=T9."Enabled" ("Disabled")) -> ()  [unwired: 2 in, 2 out]
      n201 = call "Capacity.vi"("Exit"=TRUE, "NI1"=w382, "NI2"=w381) -> ()  [unwired: 11 in, 2 out]
      n202 = call "DecorationVisibility.vi"("Visible"=TRUE, "TabControl in"=w377) -> ()  [unwired: 9 in, 1 out]
    }
    frame #5 {
      n203 = disable-structure shown="Enabled" {
        frame Disabled {
          n204 = control-ref of="This VI"() -> (w383:refnum<vi>)
          n205 = invoke class="VI" method="FP.Close"(reference=w383) -> ()  [unwired: 2 in, 3 out]
        }
        frame Enabled {
        }
      }
    }
  }
